vi "FTW-JSON-Format-String.vi"(1 "LabVIEW String":string) -> (0 "JSON String":string)   [LabVIEW 2012]
panel:
  # "Inputs"
  # "Outputs"
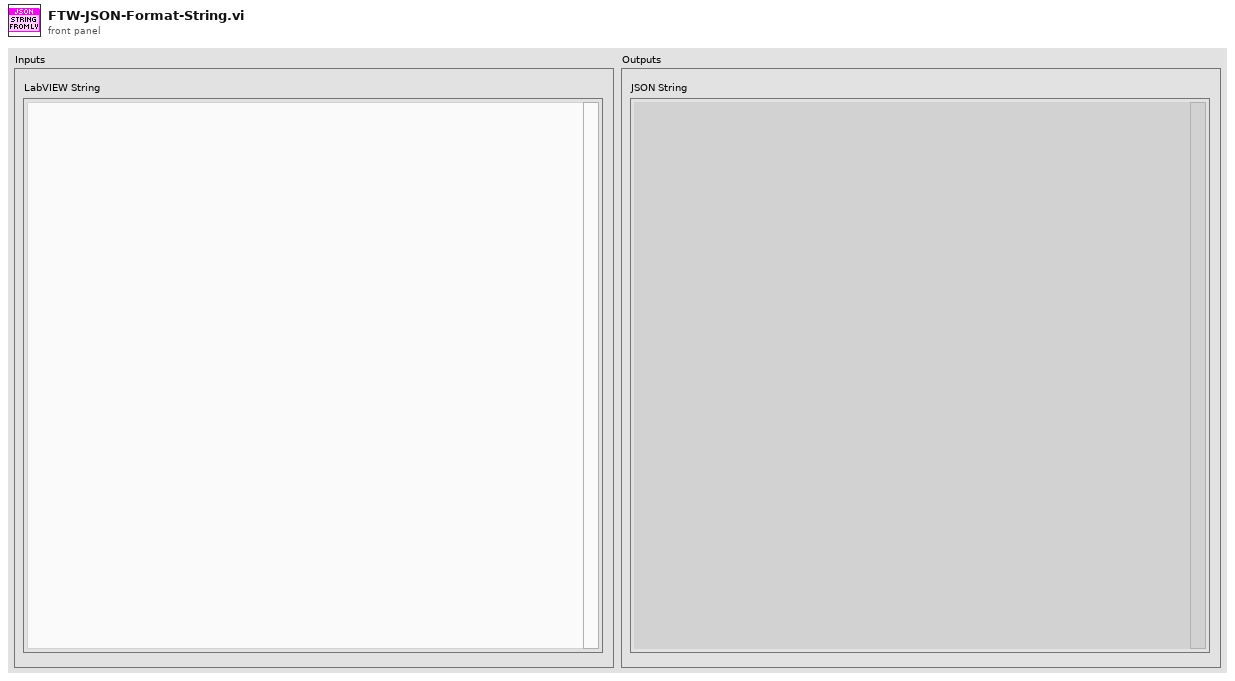
[diagram p1: front panel]
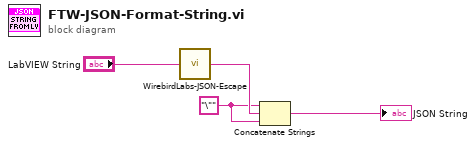
[diagram p0: block diagram]
diagram:
  w1 = "\"" ("string")
  n1 = call "WirebirdLabs-JSON-Escape.vi"("String"="LabVIEW String") -> ("Escaped String"=w3:string)
  n2 = Concatenate Strings(w1, w3, w1) -> (→"JSON String":string)
